vi "Abort.vi"(8 "error in (no error)":errorcluster, 11 "DeployResource in":refnum<class "DeployResource.lvclass">) -> (0 "error out":errorcluster, 2 "Stopped?":bool, 3 "DeployResource out":refnum<class "DeployResource.lvclass">, 5 "Returned Data":string)   [LabVIEW 2020, in "PicoG-Core.lvlib" / "DeployResource.lvclass"]
uses:
  DeployResource.lvclass
panel:
  # "Can remove this later.\nNow, it helps with error debug."
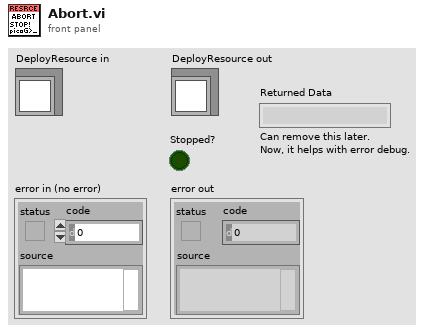
[diagram p1: front panel]
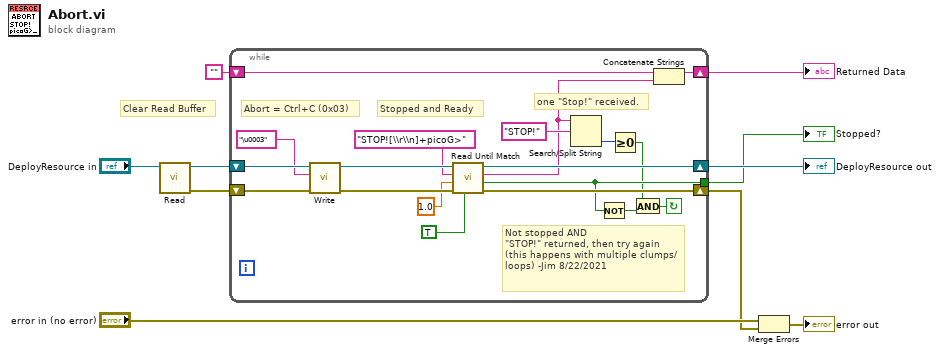
[diagram p0: block diagram]
diagram:
  # "Clear Read Buffer"
  n1 = call-dynamic "Read.vi"("DeployResource in"="DeployResource in") -> ("error out"=w7:errorcluster, "DeployResource out"=w6:refnum<class "DeployResource.lvclass">)  [unwired: 7 in, 2 out]
  n2 = while {
    tunnel: [w19] -> w3
    shift-right: [w23] -> w4
    shift-left: w7 -> [w29]
    shift-right: [w25] -> w5
    shift-left: w6 -> [w28]
    shift-right: [w14] -> w1
    shift-left: "" -> [w12]
    stop <- w15 continue-if-true
    # "Stopped and Ready"
    # "Abort = Ctrl+C (0x03)"
    # "one \"Stop!\" received."
    # "Not stopped AND\n\"STOP!\" returned, then try again\n(this happens with multiple clumps/loops) -Jim 8/22/2021"
    n3 = call-dynamic "Write.vi"("error in (no error)"=w29, "Data"="\u0003", "DeployResource in"=w28) -> ("error out"=w24:errorcluster, "DeployResource out"=w26:refnum<class "DeployResource.lvclass">)  [unwired: 6 in, 1 out]
    n4 = call "Read Until Match.vi"("Regular Expression?"=TRUE, "error in (no error)"=w24, "Timeout S (0)"=1.0, "Match String"="STOP![\\r\\n]+picoG>", "DeployResource in"=w26) -> ("error out"=w23:errorcluster, "Found?"=w19:bool, "Data"=w13:string, "DeployResource out"=w25:refnum<class "DeployResource.lvclass">)  [unwired: 3 in]
    n5 = Search/Split String(string=w13, search string/char (-)="STOP!" ("Match String")) -> (offset of match=w17:i32)  [unwired: 1 in, 2 out]
    n6 = Not(x=w19) -> (.not. x?=w18:bool)
    n7 = Greater Or Equal To 0?(x=w17) -> (x >= 0?=w16:bool)
    n8 = And(x=w16, y=w18) -> (x .and. y?=w15:bool)
    n9 = Concatenate Strings(w12, w13) -> (w14:string)
  }
  "DeployResource out" <- w5
  "Stopped?" <- w3
  "Returned Data" <- w1
  n10 = Merge Errors("error in (no error)", w4) -> (→"error out":errorcluster)
